vi "ReadFile_funzioni_correttrici.vi"() -> (2 "Contenuto file":string[][](array[string]))   [LabVIEW 2019]
uses:
  <vilib>/Utility/file.llb/Read Delimited Spreadsheet (string).vi
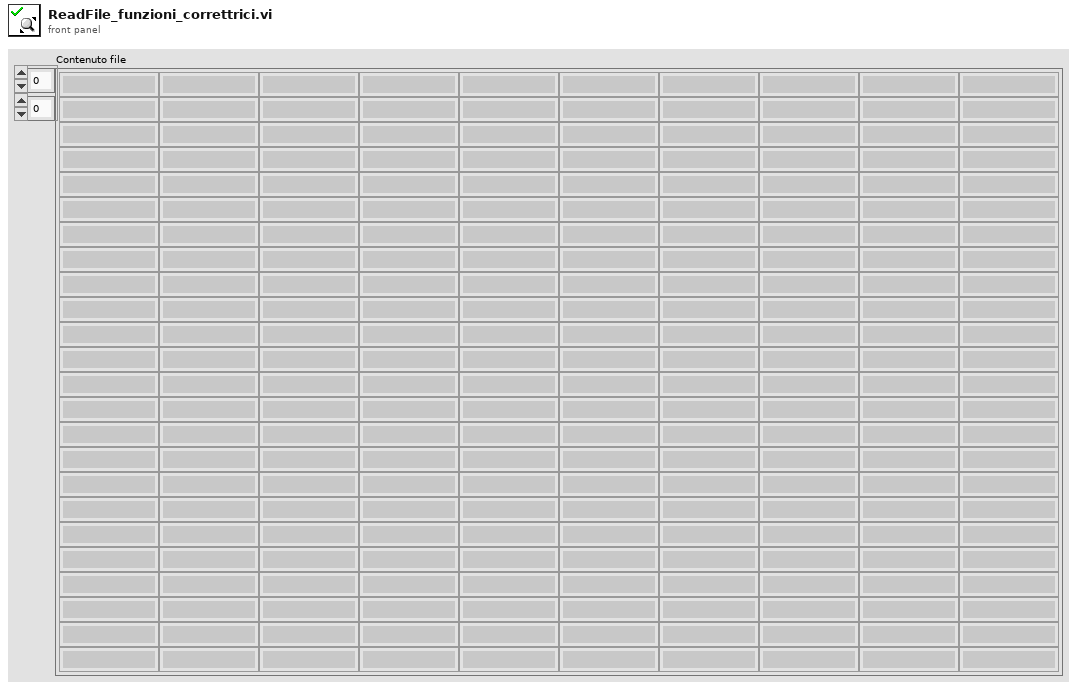
[diagram p1: front panel]
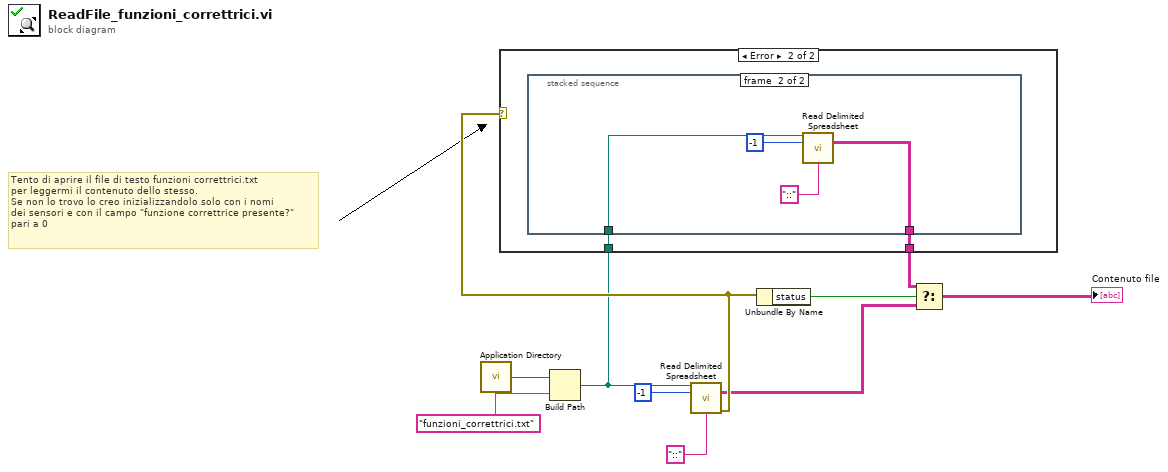
[diagram p0: block diagram]
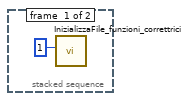
[diagram p3: hidden frame]
diagram:
  # "Tento di aprire il file di testo funzioni correttrici.txt\nper leggermi il contenuto dello stesso. \nSe non lo trovo lo creo inizializzandolo solo con i nomi \ndei sensori e con il campo \"funzione correttrice presente?\"\npari a 0"
  n1 = call <vilib>:"Application Directory.vi"() -> ("Application Directory"=w9:path)
  n2 = Build Path(base path=w9, name or relative path="funzioni_correttrici.txt") -> (appended path=w1:path)
  n3 = call-poly <vilib>:"Read Delimited Spreadsheet.vi"("file path (dialog if empty)"=w1, "number of rows (all:-1)"=-1, "delimiter (\\t)"="::" ("delimiter (\\t)")) -> ("all rows"=w5:string[][], "error out"=w7:errorcluster)  [unwired: 7 in, 4 out]
  n4 = case shown="Error" w7 {
    tunnel: [_ w12] -> w6
    tunnel: w1 -> [_ w11]
    frame No Error {
    }
    frame Error {
      n5 = stacked-sequence {
        tunnel: [_ w15] -> w12
        tunnel: w11 -> [_ w14]
        frame #0 {
          n6 = call "InizializzaFile_funzioni_correttrici.vi"("banco"=1) -> ()  [unwired: 11 in]
        }
        frame #1 {
          n7 = call-poly <vilib>:"Read Delimited Spreadsheet.vi"("file path (dialog if empty)"=w14, "number of rows (all:-1)"=-1, "delimiter (\\t)"="::" ("delimiter (\\t)")) -> ("all rows"=w15:string[][])  [unwired: 7 in, 5 out]
        }
      }
    }
  }
  n8 = Unbundle By Name(w7) -> ("status"=w4:bool)
  n9 = Select(t=w6, s=w4, f=w5) -> (s? t:f=→"Contenuto file":string[][])
